vi "12_19_Fxp_addation.vi"(1 "y":fxp<+/-,19,12>, 2 "x":fxp<+/-,19,12>) -> (0 "x+y":fxp<+/-,20,13> format="%.41g")   [LabVIEW 2020]
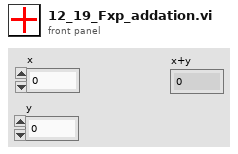
[diagram p1: front panel]
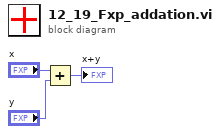
[diagram p0: block diagram]
diagram:
  n1 = Add(x="x", y="y") -> (x+y=→"x+y":fxp<+/-,20,13>)
